vi "LDR İLE SAYDAMLIK ÖLÇÜMÜ.vi"() -> ()   [LabVIEW 2017]
doc: "Measure light intensity using a photocell."
uses:
  <vilib>/MakerHub/LINX/Public/Peripherals/Digital/Digital Write 1 Chan.vi
  <vilib>/MakerHub/LINX/Public/Peripherals/Digital/Digital Write N Chans.vi
  <vilib>/MakerHub/LINX/Private/Local IO/LinxDigitalWrite.vi
  <vilib>/MakerHub/LINX/Public/Utilities/Check Channel.vi
  <vilib>/MakerHub/LINX/Public/Utilities/Open Serial.vi
  <vilib>/MakerHub/LINX/Private/Utilties/Generate Error.vi
  <vilib>/MakerHub/LINX/LMH-LINX.lvlib
panel:
  out "LDR Değeri":u8(slide) scale=0.0..50.0
  in  "ANALOG KANALI":u8
  in  "PORT SEÇİNİZ":refnum<visa-resource-name>
  in  "Stop Button":bool
  # "LDR"
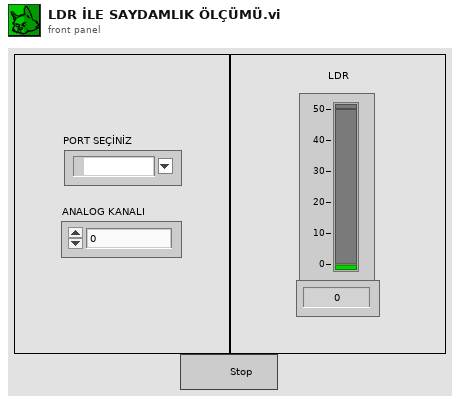
[diagram p1: front panel]
types:
  T1 = typedef "LMH-LINX.lvlib/LINX Ref.ctl" = cluster{"IO":T2, "Interface":T3, "LINX Device Config":T4}
  T2 = typedef "LMH-LINX.lvlib/Platform.ctl" = enum16{"Remote", "Local"}
  T3 = typedef "LMH-LINX.lvlib/Interface.ctl" = enum16{"Serial", "TCP"}
  T4 = typedef "LMH-LINX.lvlib/Device.lvlib/LINX Device Config.ctl" = cluster{"Interface":T3, "COM Port":refnum<visa-resource-name>, "TCP Configuration":T5, "Device Family":u8, "Device ID":u8, "Device Name":string, "TCP Ref":refnum<k5>, "Channels":T6}
  T5 = typedef "LMH-LINX.lvlib/Device.lvlib/TCP Config.ctl" = cluster{"IP Address":string, "Port":u16}
  T6 = typedef "LMH-LINX.lvlib/Channels.ctl" = cluster{"DI":u8[], "DO":u8[], "AI":u8[], "AO":u8[], "PWM":u8[], "QE":u8[], "UART":u8[], "I2C 2":u8[], "SPI":u8[], "CAN":u8[], "Servo":u8[], "AI Ref (V)":dbl, "AI Resolution (Bits)":u8, "AO Ref (V)":dbl, "AO Resolution (Bits)":u8}
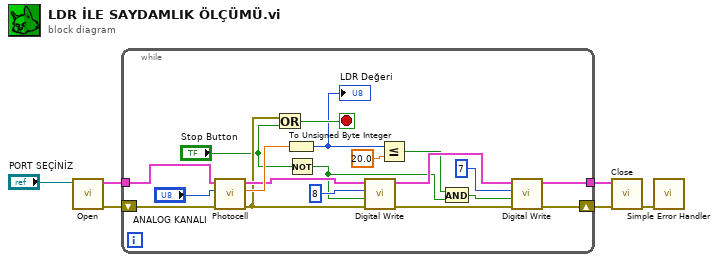
[diagram p0: block diagram]
diagram:
  n1 = call-poly <vilib>:"Open.vi"("Serial Port"="PORT SEÇİNİZ") -> ("Error Out"=w5:errorcluster, "LINX Resource"=w6:T1)  [unwired: 8 in, 1 out]
  n2 = while {
    tunnel: w6 -> [w24]
    tunnel: [w16] -> w4
    shift-right: [w15] -> w3
    shift-left: w5 -> [w23]
    stop <- w25 stop-if-true
    n3 = call <vilib>:"Photocell.vi"("Error In"=w23, "AI Channel"="ANALOG KANALI", "LINX Resource"=w24) -> ("Error Out"=w19:errorcluster, "Value (0-100)"=w21:dbl, "LINX Resource"=w20:T1)  [unwired: 6 in]
    n4 = Or(x=w19, y="Stop Button") -> (x .or. y?=w25:bool)
    n5 = To Unsigned Byte Integer(number=w21) -> (unsigned 8bit integer=w10:u8)
    "LDR Değeri" <- w10
    n6 = Not(x="Stop Button") -> (.not. x?=w8:bool)
    n7 = call-poly <vilib>:"Digital Write.vi"("Error In"=w19, "Output Value"=w8, "DO Channel"=u8 8, "LINX Resource"=w20) -> ("Error Out"=w14:errorcluster, "LINX Resource"=w13:T1)  [unwired: 6 in]
    n8 = Less Or Equal?(x=w10, y=20.0) -> (x <= y?=w9:bool)
    n9 = And(x=w9, y=w8) -> (x .and. y?=w7:bool)
    n10 = call-poly <vilib>:"Digital Write.vi"("Error In"=w14, "Output Value"=w7, "DO Channel"=u8 7, "LINX Resource"=w13) -> ("Error Out"=w15:errorcluster, "LINX Resource"=w16:T1)  [unwired: 6 in]
  }
  n11 = call <vilib>:"Close.vi"("Error In"=w3, "LINX Resource"=w4) -> ("Error Out"=w1:errorcluster)  [unwired: 9 in]
  n12 = call <vilib>:"Simple Error Handler.vi"("error in (no error)"=w1) -> ()  [unwired: 4 in, 5 out]
